vi "Pre Launch Init.vi"(11 "Camera_Controller in":refnum<class "Camera_Controller.lvclass">) -> (0 "error out":errorcluster, 3 "Camera_Controller out":refnum<class "Camera_Controller.lvclass">)   [LabVIEW 2023, in "Camera_Controller.lvlib" / "Camera_Controller.lvclass"]
doc: "(<B>Filename</B>: Actor Framework.lvlib:Actor.lvclass:Pre Launch Init.vi)\n\nDefines behavior that occurs after the Launch Nested Actor method is invoked but before the actor's Actor Core method begins running.\n\nBy default, this method does nothing. A descendant class may override it to define behavior."
uses:
  Camera_Controller.lvclass
  <vilib>/vision/Image Controls.llb/IMAQ Image.ctl
  Camera_Controller.lvclass/Camera_Controller.ctl
  <vilib>/ActorFramework/Actor/Actor.lvclass
panel:
  in  "Instruments Found":T1
  in  "Variant":variant
  in  "Exposure(ms)":dbl
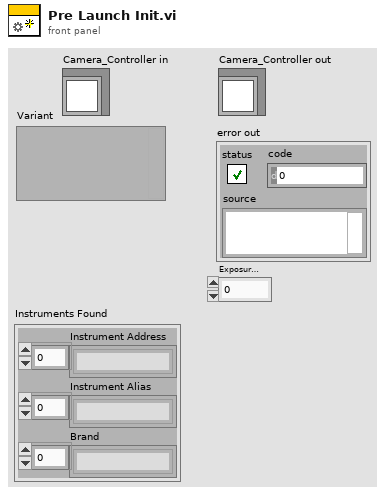
[diagram p1: front panel]
types:
  T1 = cluster{"Instrument Address":string[], "Instrument Alias":string[], "Brand":string[]}
  T2 = typedef "IMAQ Image.ctl" = refnum<image>
  T3 = cluster{"Image In":T2, "Processed Frames per Second":dbl}
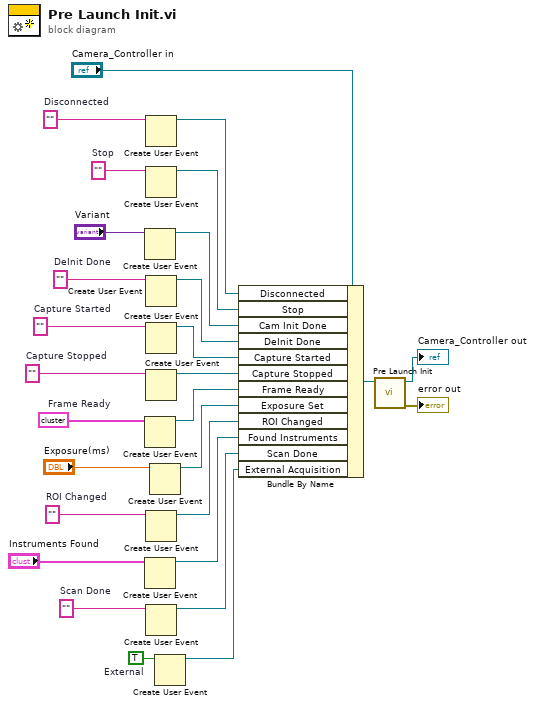
[diagram p0: block diagram]
diagram:
  w2 = TRUE  # External
  w4 = ""  # Scan Done
  w6 = ""  # Disconnected
  w12 = ""  # ROI Changed
  w16 = T3 {"Image In"=refnum, "Processed Frames per Second"=0.0}  # Frame Ready
  w18 = ""  # Capture Stopped
  w20 = ""  # Capture Started
  w22 = ""  # DeInit Done
  w23 = ""  # Stop
  n1 = Create User Event(user event datatype="Variant") -> (user event=w9:refnum<user-event>)  [unwired: 1 in, 1 out]
  n2 = Create User Event(user event datatype=w16) -> (user event=w15:refnum<user-event>)  [unwired: 1 in, 1 out]
  n3 = Create User Event(user event datatype="Instruments Found") -> (user event=w8:refnum<user-event>)  [unwired: 1 in, 1 out]
  n4 = Create User Event(user event datatype=w6) -> (user event=w5:refnum<user-event>)  [unwired: 1 in, 1 out]
  n5 = Create User Event(user event datatype=w23) -> (user event=w24:refnum<user-event>)  [unwired: 1 in, 1 out]
  n6 = Create User Event(user event datatype=w22) -> (user event=w21:refnum<user-event>)  [unwired: 1 in, 1 out]
  n7 = Create User Event(user event datatype=w20) -> (user event=w19:refnum<user-event>)  [unwired: 1 in, 1 out]
  n8 = Create User Event(user event datatype=w18) -> (user event=w17:refnum<user-event>)  [unwired: 1 in, 1 out]
  n9 = Create User Event(user event datatype=w12) -> (user event=w11:refnum<user-event>)  [unwired: 1 in, 1 out]
  n10 = Create User Event(user event datatype=w4) -> (user event=w3:refnum<user-event>)  [unwired: 1 in, 1 out]
  n11 = Create User Event(user event datatype="Exposure(ms)") -> (user event=w13:refnum<user-event>)  [unwired: 1 in, 1 out]
  n12 = Create User Event(user event datatype=w2) -> (user event=w1:refnum<user-event>)  [unwired: 1 in, 1 out]
  n13 = Bundle By Name(cluster="Camera_Controller in", "Disconnected"=w5, "Stop"=w24, "Cam Init Done"=w9, "DeInit Done"=w21, "Capture Started"=w19, "Capture Stopped"=w17, "Frame Ready"=w15, "Exposure Set"=w13, "ROI Changed"=w11, "Found Instruments"=w8, "Scan Done"=w3, "External Acquisition"=w1) -> (w25:refnum<class "Camera_Controller.lvclass">)
  n14 = call-parent "Pre Launch Init.vi"("Actor in"=w25) -> ("error out"=→"error out":errorcluster, "Actor out"=→"Camera_Controller out":refnum<class "Camera_Controller.lvclass">)  [unwired: 9 in]
